vi "test report api.vi"() -> ()   [LabVIEW 2019]
uses:
  <vilib>/Utility/sysdir.llb/System Directory Type.ctl
  <vilib>/httpClient/POSTBuffer.vi
  <userlib>/_OpenG.lib/array/array.llb/Remove Duplicates from 1D Array (String)__ogtk.vi
  <userlib>/_OpenG.lib/array/array.llb/Delete Elements from 1D Array (String)__ogtk.vi
  <vilib>/httpClient/LabVIEWHTTPClient.lvlib
panel:
  out "body 4":string
  out "JSON string 3":string
  out "data":string[][](array[string])
  out "body 3":string
  out "JSON string 2":string
  out "Table Control":string[][](table)
  out "value":T1
  out "body 2":string
  out "testname":string[](array[string])
  out "testtype":string[](array[string])
  out "JSON string":string
  out "body":string
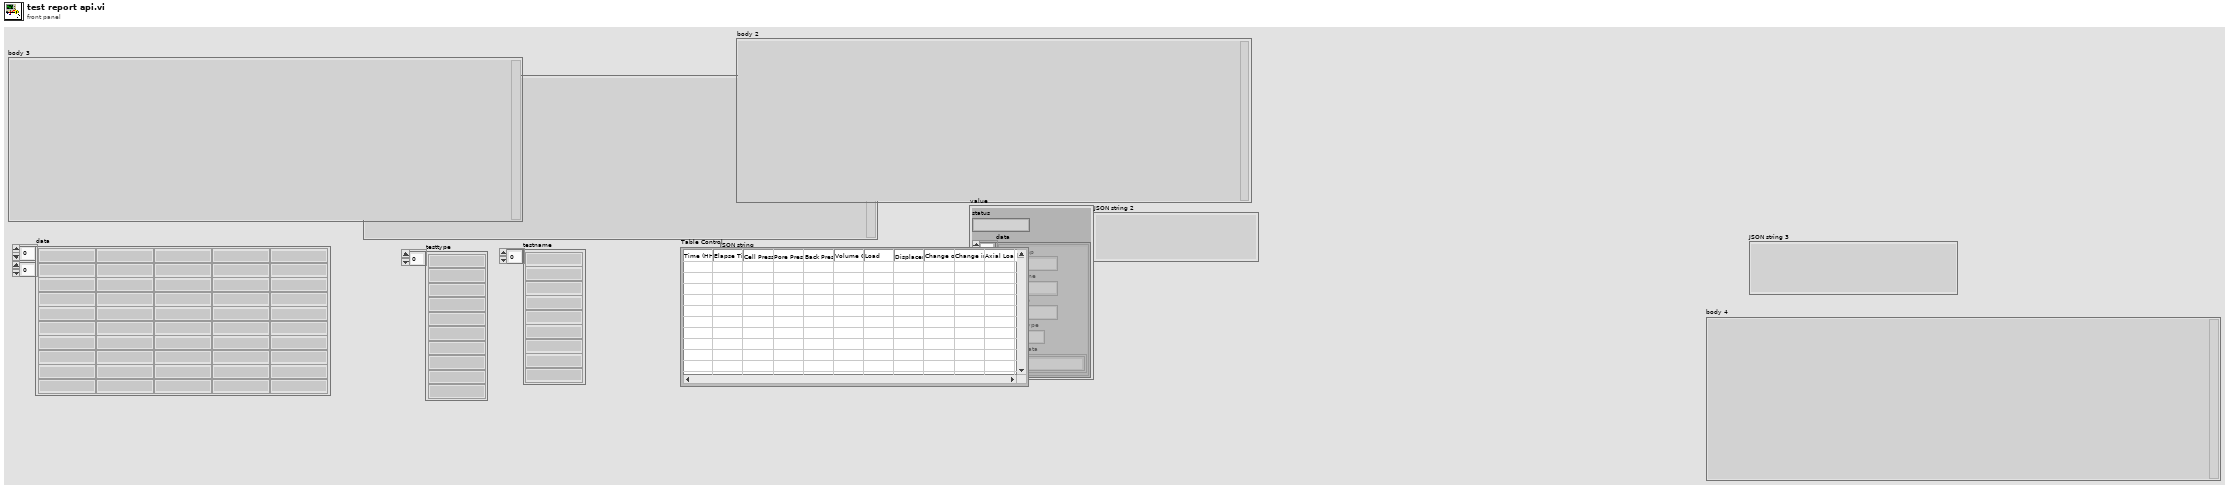
[diagram p1: front panel]
types:
  T1 = cluster{"status":string, "data":cluster{"timestamp":string, "elapsetime":string, "testname":string, "testtype":u16, "data":string[]}[]}
  T2 = cluster{"status":string, "data":cluster{"id":string, "testname":string, "jobno":string, "jobdesc":string, "sampleid":string, "date":string}[]}
  T3 = typedef "System Directory Type.ctl" = i32
  T4 = enum16{"open", "open or create", "create or replace", "create", "open (read-only)"}
  T5 = cluster{"status":string, "data":cluster{"testname":string, "testtype":string}[]}
  T6 = typedef "LabVIEWHTTPClient.lvlib/ClientHandle.ctl" = refnum<k1>
  T7 = cluster{"id":string, "testname":string, "jobno":string, "jobdesc":string, "sampleid":string, "date":string}[]
  T8 = cluster{"testtype":u16, "testname":string, "fileid":string}
  T9 = cluster{"timestamp":string, "elapsetime":string, "testname":string, "testtype":u16, "data":string[]}[]
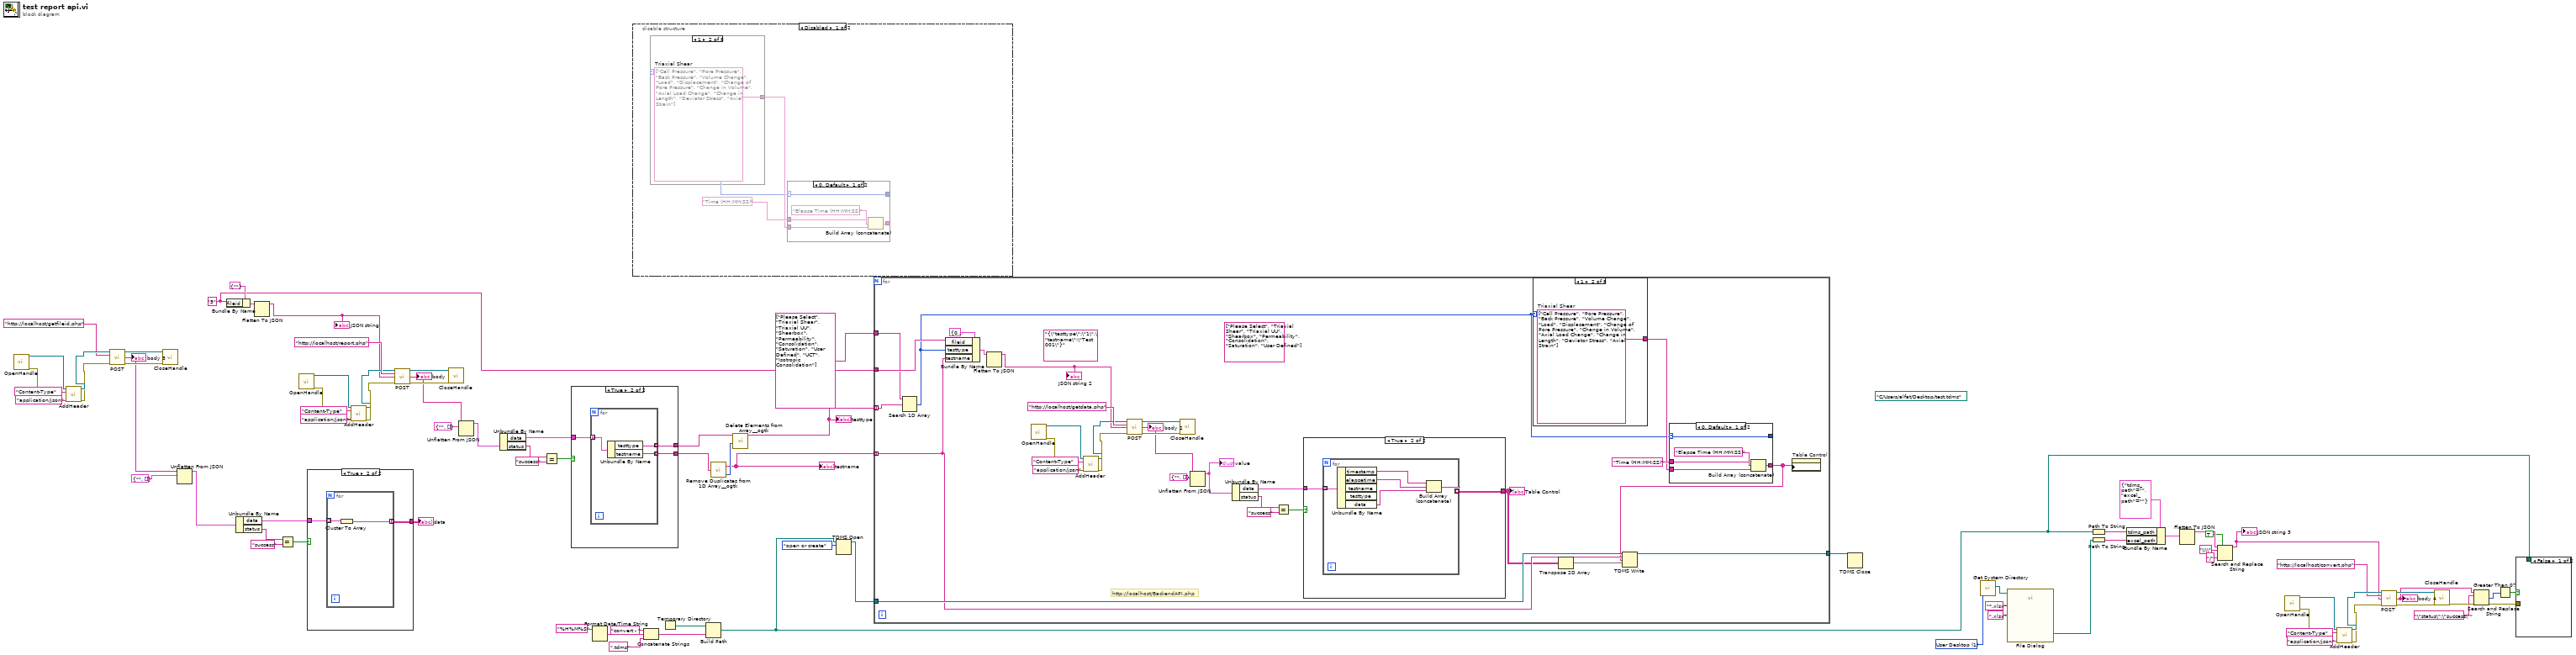
[diagram p0: block diagram]
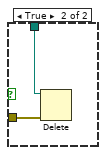
[diagram p2: hidden frame]
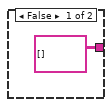
[diagram p3: hidden frame]
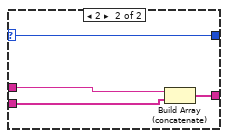
[diagram p4: hidden frame]
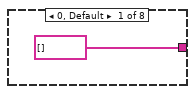
[diagram p5: hidden frame]
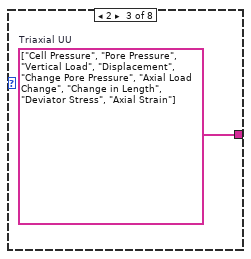
[diagram p6: hidden frame]
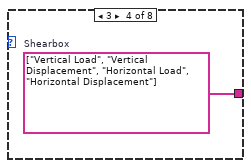
[diagram p7: hidden frame]
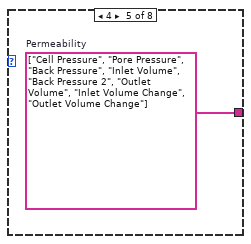
[diagram p8: hidden frame]
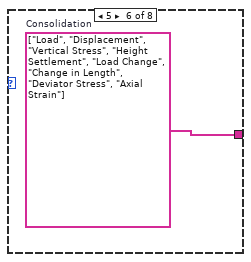
[diagram p9: hidden frame]
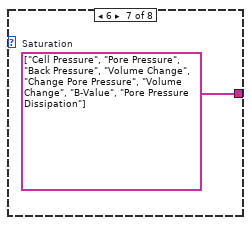
[diagram p10: hidden frame]
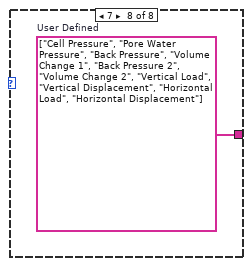
[diagram p11: hidden frame]
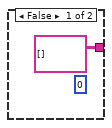
[diagram p12: hidden frame]
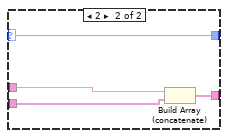
[diagram p13: hidden frame]
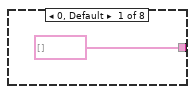
[diagram p14: hidden frame]
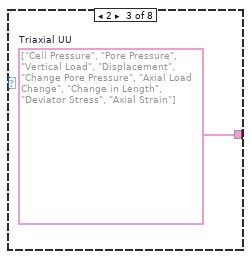
[diagram p15: hidden frame]
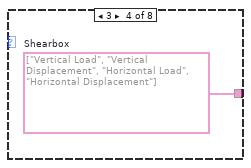
[diagram p16: hidden frame]
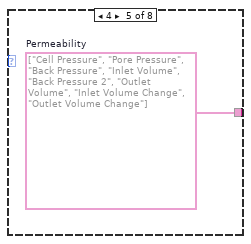
[diagram p17: hidden frame]
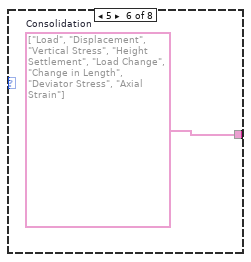
[diagram p18: hidden frame]
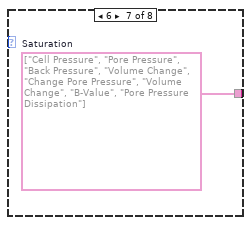
[diagram p19: hidden frame]
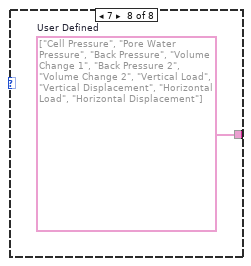
[diagram p20: hidden frame]
diagram:
  (unwired) path "C:/Users/alfat/Desktop/test.tdms"
  w52 = T3 1 items=["User Home"=0, "User Desktop"=1, "User Documents"=2, "User Application Data"=3, "User Preferences"=4, "User Temporary"=5, "Public Documents"=6, "Public Application Data"=7, "Public Preferences"=8, "Public Cache"=13, "System Core Libraries"=9, "System Installed Libraries"=10, "Application Files"=11, "Boot Volume Root"=12] ("system directory type")
  w58 = "5" ("fileid")
  n1 = call <vilib>:"OpenHandle.vi"() -> ("client handle out"=w46:T6, "error out"=w44:errorcluster)  [unwired: 14 in]
  n2 = call <vilib>:"AddHeader.vi"("client handle"=w46, "header"="Content-Type", "value"="application/json", "error in (no error)"=w44) -> ("client handle out"=w47:T6, "error out"=w45:errorcluster)  [unwired: 10 in]
  n3 = call-poly <vilib>:"POST.vi"("client handle"=w47, "url"="http://localhost/getfileid.php", "error in (no error)"=w45) -> ("client handle out"=w42:T6, "body"=w39:string, "error out"=w41:errorcluster)  [unwired: 9 in, 1 out]
  "body 3" <- w39
  n4 = call <vilib>:"CloseHandle.vi"("client handle"=w42, "error in (no error)"=w41) -> ()  [unwired: 13 in, 1 out]
  n5 = Unflatten From JSON(JSON string=w39, type and defaults=T2 {"status"="", "data"=[]}) -> (value=w34:T2)  [unwired: 5 in, 1 out]
  n6 = Bundle By Name(cluster=cluster{"fileid":string} {"fileid"=""}, "fileid"=w58) -> (w65:cluster{"fileid":string})
  n7 = Unbundle By Name(w34) -> ("data"=w38:T7, "status"=w35:string)
  n8 = Flatten To JSON(anything=w65) -> (JSON string=w64:string)  [unwired: 2 in, 1 out]
  "JSON string" <- w64
  n9 = Equal?(x=w35, y="success") -> (x = y?=w37:bool)
  n10 = call <vilib>:"OpenHandle.vi"() -> ("client handle out"=w77:T6, "error out"=w79:errorcluster)  [unwired: 14 in]
  n11 = case shown="True" w37 {
    tunnel: w38 -> [_ w85]
    tunnel: [string[][] [] ("data") w84] -> w33
    frame False {
    }
    frame True {
      n12 = for {
        tunnel: w85 -> [w87] mode=indexing
        tunnel: [w86] -> w84 mode=indexing
        n13 = Cluster To Array(cluster=w87) -> (array=w86:string[])
      }
    }
  }
  "data" <- w33
  n14 = call <vilib>:"AddHeader.vi"("client handle"=w77, "header"="Content-Type", "value"="application/json", "error in (no error)"=w79) -> ("client handle out"=w76:T6, "error out"=w78:errorcluster)  [unwired: 10 in]
  n15 = call-poly <vilib>:"POST.vi"("client handle"=w76, "url"="http://localhost/report.php", "buffer"=w64, "error in (no error)"=w78) -> ("client handle out"=w81:T6, "body"=w73:string, "error out"=w82:errorcluster)  [unwired: 8 in, 1 out]
  "body" <- w73
  n16 = call <vilib>:"CloseHandle.vi"("client handle"=w81, "error in (no error)"=w82) -> ()  [unwired: 13 in, 1 out]
  n17 = Unflatten From JSON(JSON string=w73, type and defaults=T5 {"status"="", "data"=[]}) -> (value=w71:T5)  [unwired: 5 in, 1 out]
  n18 = Unbundle By Name(w71) -> ("data"=w67:cluster{"testname":string, "testtype":string}[], "status"=w70:string)
  n19 = Equal?(x=w70, y="success") -> (x = y?=w68:bool)
  n20 = case shown="True" w68 {
    tunnel: w67 -> [_ w92]
    tunnel: [string[] [] w91] -> w62
    tunnel: [string[] [] w90] -> w63
    frame False {
    }
    frame True {
      n21 = for {
        tunnel: w92 -> [w95] mode=indexing
        tunnel: [w94] -> w91 mode=indexing
        tunnel: [w93] -> w90 mode=indexing
        n22 = Unbundle By Name(w95) -> ("testtype"=w94:string, "testname"=w93:string)
      }
    }
  }
  n23 = Format Date/Time String(time format string (%c)="%H%M%S") -> (date/time string=w12:string)  [unwired: 2 in]
  n24 = disable-structure shown="Disabled" {
    frame Disabled {
      n25 = case shown="1" w97 {
        tunnel: [string[] [] w110 w111 w112 w113 w114 w115 w116] -> w98
        frame 0, Default {
        }
        frame 1 {
          w110 = string[] ["Cell Pressure", "Pore Pressure", "Back Pressure", "Volume Change", "Load", "Displacement", "Change of Pore Pressure", "Change in Volume", "Axial Load Change", "Change in Length", "Deviator Stress", "Axial Strain"]  # Triaxial Shear
        }
        frame 2 {
          w111 = string[] ["Cell Pressure", "Pore Pressure", "Vertical Load", "Displacement", "Change Pore Pressure", "Axial Load Change", "Change in Length", "Deviator Stress", "Axial Strain"]  # Triaxial UU
        }
        frame 3 {
          w112 = string[] ["Vertical Load", "Vertical Displacement", "Horizontal Load", "Horizontal Displacement"]  # Shearbox
        }
        frame 4 {
          w113 = string[] ["Cell Pressure", "Pore Pressure", "Back Pressure", "Inlet Volume", "Back Pressure 2", "Outlet Volume", "Inlet Volume Change", "Outlet Volume Change"]  # Permeability
        }
        frame 5 {
          w114 = string[] ["Load", "Displacement", "Vertical Stress", "Height Settlement", "Load Change", "Change in Length", "Deviator Stress", "Axial Strain"]  # Consolidation
        }
        frame 6 {
          w115 = string[] ["Cell Pressure", "Pore Pressure", "Back Pressure", "Volume Change", "Change Pore Pressure", "Volume Change", "B-Value", "Pore Pressure Dissipation"]  # Saturation
        }
        frame 7 {
          w116 = string[] ["Cell Pressure", "Pore Water Pressure", "Back Pressure", "Volume Change 1", "Back Pressure 2", "Volume Change 2", "Vertical Load", "Vertical Displacement", "Horizontal Load", "Horizontal Displacement"]  # User Defined
        }
      }
      n26 = case shown="0, Default" w97 {
        selector: w97 -> [w100 w105]
        tunnel: "Time (HH:MM:SS)" ("element") -> [w103 w108]
        tunnel: w98 -> [w102 w107]
        tunnel: [w101 w106] -> w96
        tunnel: [w100 w105] -> _
        frame 0, Default {
          n27 = Build Array (concatenate)(w103, "Elapse Time (HH:MM:SS)" ("String"), w102) -> (w101:string[])
        }
        frame 2 {
          n28 = Build Array (concatenate)(w108, w107) -> (w106:string[])
        }
      }
    }
    frame Enabled {
    }
  }
  n29 = Concatenate Strings("convert - " ("string"), w12, ".tdms" ("string")) -> (w9:string)
  n30 = Temporary Directory() -> (w10:path)
  n31 = Build Path(base path=w10, name or relative path=w9) -> (appended path=w7:path)
  n32 = call-poly <userlib>:"Remove Duplicates from 1D Array__ogtk.vi"("Input Array"=w63) -> ("Output Array"=w59:string[], "indices of removed elements"=w61:i32[])
  "testname" <- w59
  n33 = call-poly <userlib>:"Delete Elements from Array__ogtk.vi"("indices"=w61, "array"=w62) -> ("array w/ subset deleted"=w60:string[])  [unwired: 8 in, 1 out]
  "testtype" <- w60
  n34 = TDMS Open(10:T4."open or create" ("operation (0:open)"), 11:w7) -> (3:w55:refnum<k34>)  [unwired: 5 in, 1 out]
  n35 = for {
    tunnel: w60 -> [w125] mode=indexing
    tunnel: w59 -> [w121] mode=indexing
    tunnel: w58 -> [w126]
    tunnel: string[] ["Please Select", "Triaxial Shear", "Triaxial UU", "Shearbox", "Permeability", "Consolidation", "Saturation", "User Defined", "UCT", "Isotropic Consolidation"] ("Strings []") -> [w124]
    tunnel: w55 -> [w122]
    tunnel: [w118] -> w54
    (unwired) string[] ["Please Select", "Triaxial Shear", "Triaxial UU", "Shearbox", "Permeability", "Consolidation", "Saturation", "User Defined"] ("Strings []")
    (unwired) "{\"testtype\":\"1\",\"testname\":\"Test 001\"}" ("buffer")
    # "http://localhost/BackendAPI.php"
    n36 = Search 1D Array(1D array=w124, element=w125) -> (index of element=w123:i32)  [unwired: 1 in]
    n37 = Bundle By Name(cluster=T8 {"testtype"=0, "testname"="", "fileid"=""}, "fileid"=w126, "testtype"=w123, "testname"=w121) -> (w130:T8)
    n38 = Flatten To JSON(anything=w130) -> (JSON string=w129:string)  [unwired: 2 in, 1 out]
    "JSON string 2" <- w129
    n39 = call <vilib>:"OpenHandle.vi"() -> ("client handle out"=w142:T6, "error out"=w144:errorcluster)  [unwired: 14 in]
    n40 = call <vilib>:"AddHeader.vi"("client handle"=w142, "header"="Content-Type", "value"="application/json", "error in (no error)"=w144) -> ("client handle out"=w141:T6, "error out"=w143:errorcluster)  [unwired: 10 in]
    n41 = call-poly <vilib>:"POST.vi"("client handle"=w141, "url"="http://localhost/getdata.php", "buffer"=w129, "error in (no error)"=w143) -> ("client handle out"=w146:T6, "body"=w138:string, "error out"=w147:errorcluster)  [unwired: 8 in, 1 out]
    "body 2" <- w138
    n42 = call <vilib>:"CloseHandle.vi"("client handle"=w146, "error in (no error)"=w147) -> ()  [unwired: 13 in, 1 out]
    n43 = Unflatten From JSON(JSON string=w138, type and defaults=T1 {"status"="", "data"=[]}) -> (value=w136:T1)  [unwired: 5 in, 1 out]
    "value" <- w136
    n44 = Unbundle By Name(w136) -> ("data"=w132:T9, "status"=w135:string)
    n45 = Equal?(x=w135, y="success") -> (x = y?=w133:bool)
    n46 = case shown="True" w133 {
      tunnel: w132 -> [_ w167]
      tunnel: [string[][] [] w166] -> w119
      frame False {
        (unwired) u16 0 ("testtype")
      }
      frame True {
        n47 = for {
          tunnel: w167 -> [w172] mode=indexing
          tunnel: [w168] -> w166 mode=indexing
          n48 = Unbundle By Name(w172) -> ("timestamp"=w171:string, "elapsetime"=w170:string, "data"=w169:string[])  [unwired: 2 out]
          n49 = Build Array (concatenate)(w171, w170, w169) -> (w168:string[])
        }
      }
    }
    "Table Control" <- w119
    n50 = case shown="1" w123 {
      tunnel: [string[] [] w158 w159 w160 w161 w162 w163 w164] -> w127
      frame 0, Default {
      }
      frame 1 {
        w158 = string[] ["Cell Pressure", "Pore Pressure", "Back Pressure", "Volume Change", "Load", "Displacement", "Change of Pore Pressure", "Change in Volume", "Axial Load Change", "Change in Length", "Deviator Stress", "Axial Strain"]  # Triaxial Shear
      }
      frame 2 {
        w159 = string[] ["Cell Pressure", "Pore Pressure", "Vertical Load", "Displacement", "Change Pore Pressure", "Axial Load Change", "Change in Length", "Deviator Stress", "Axial Strain"]  # Triaxial UU
      }
      frame 3 {
        w160 = string[] ["Vertical Load", "Vertical Displacement", "Horizontal Load", "Horizontal Displacement"]  # Shearbox
      }
      frame 4 {
        w161 = string[] ["Cell Pressure", "Pore Pressure", "Back Pressure", "Inlet Volume", "Back Pressure 2", "Outlet Volume", "Inlet Volume Change", "Outlet Volume Change"]  # Permeability
      }
      frame 5 {
        w162 = string[] ["Load", "Displacement", "Vertical Stress", "Height Settlement", "Load Change", "Change in Length", "Deviator Stress", "Axial Strain"]  # Consolidation
      }
      frame 6 {
        w163 = string[] ["Cell Pressure", "Pore Pressure", "Back Pressure", "Volume Change", "Change Pore Pressure", "Volume Change", "B-Value", "Pore Pressure Dissipation"]  # Saturation
      }
      frame 7 {
        w164 = string[] ["Cell Pressure", "Pore Water Pressure", "Back Pressure", "Volume Change 1", "Back Pressure 2", "Volume Change 2", "Vertical Load", "Vertical Displacement", "Horizontal Load", "Horizontal Displacement"]  # User Defined
      }
    }
    n51 = Transpose 2D Array(2D array=w119) -> (transposed array=w117:string[][])
    n52 = case shown="0, Default" w123 {
      selector: w123 -> [w148 w153]
      tunnel: "Time (HH:MM:SS)" ("element") -> [w151 w156]
      tunnel: w127 -> [w150 w155]
      tunnel: [w149 w154] -> w120
      tunnel: [w148 w153] -> _
      frame 0, Default {
        n53 = Build Array (concatenate)(w151, "Elapse Time (HH:MM:SS)" ("String"), w150) -> (w149:string[])
      }
      frame 2 {
        n54 = Build Array (concatenate)(w156, w155) -> (w154:string[])
      }
    }
    n55 = TDMS Write(0:w122, 5:w121, 7:w120, 9:w117) -> (4:w118:refnum<k34>)  [unwired: 2 in, 3 out]
    n56 = property on="Table Control" class="Tbl (strict)"("Column Headers[]"=w120) -> ()  [unwired: 2 in, 2 out]
  }
  n57 = TDMS Close(11:w54) -> ()  [unwired: 1 in, 2 out]
  n58 = call <vilib>:"Get System Directory.vi"("system directory type"=w52) -> ("system directory"=w53:path)  [unwired: 10 in]
  n59 = call "File Dialog"("start path"=w53, "pattern (all files)"="*.xlsx", "pattern label"=".xlsx") -> ("selected path"=w8:path)  [unwired: 9 in, 3 out]
  n60 = Path To String(path=w7) -> (string=w30:string)
  n61 = Path To String(path=w8) -> (string=w29:string)
  n62 = Bundle By Name(cluster=cluster{"tdms_path":string, "excel_path":string} {"tdms_path"="", "excel_path"=""}, "tdms_path"=w30, "excel_path"=w29) -> (w31:cluster{"tdms_path":string, "excel_path":string})
  n63 = Flatten To JSON(anything=w31) -> (JSON string=w26:string)  [unwired: 2 in, 1 out]
  n64 = Search and Replace String(replace all?=TRUE ("replace all? (F)"), input string=w26, search string="\\\\", replace string="/" ("replace string (\"\")")) -> (result string=w15:string)  [unwired: 4 in, 3 out]
  "JSON string 3" <- w15
  n65 = call <vilib>:"OpenHandle.vi"() -> ("client handle out"=w21:T6, "error out"=w19:errorcluster)  [unwired: 14 in]
  n66 = call <vilib>:"AddHeader.vi"("client handle"=w21, "header"="Content-Type", "value"="application/json", "error in (no error)"=w19) -> ("client handle out"=w22:T6, "error out"=w20:errorcluster)  [unwired: 10 in]
  n67 = call-poly <vilib>:"POST.vi"("client handle"=w22, "url"="http://localhost/convert.php", "buffer"=w15, "error in (no error)"=w20) -> ("client handle out"=w17:T6, "body"=w4:string, "error out"=w16:errorcluster)  [unwired: 8 in, 1 out]
  "body 4" <- w4
  n68 = call <vilib>:"CloseHandle.vi"("client handle"=w17, "error in (no error)"=w16) -> ("error out"=w6:errorcluster)  [unwired: 13 in]
  n69 = Search and Replace String(input string=w4, search string="\"status\":\"success\"", error in=w6) -> (number of replacements=w2:i32, error out=w5:errorcluster)  [unwired: 5 in, 2 out]
  n70 = Greater Than 0?(x=w2) -> (x > 0?=w1:bool)
  n71 = case shown="False" w1 {
    tunnel: w7 -> [_ w174]
    tunnel: w5 -> [_ w173]
    frame False {
    }
    frame True {
      n72 = Delete(path (use dialog)=w174, error in=w173) -> ()  [unwired: 3 in, 3 out]
    }
  }
